vi "Generalized SVD Decomposition.vi"   [LabVIEW 2020, in "NI_AALPro.lvlib"]
doc: "Computes the generalized singular value decomposition (GSVD) of a matrix pair (<B>A</B>,<B>B</B>). The data types you wire to the <B>A</B> and <B>B</B> inputs determine the polymorphic instance to use."
uses:
  <vilib>/Analysis/NI_AALPro.lvlib
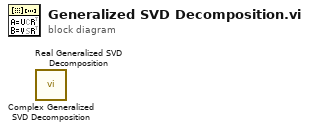
[diagram p0: block diagram]
diagram:
  n1 = call <vilib>:"Complex Generalized SVD Decomposition.vi"() -> ()  [unwired: 9 in, 7 out]
  n2 = call <vilib>:"Real Generalized SVD Decomposition.vi"() -> ()  [unwired: 9 in, 7 out]
